vi "enable channel groups.vi"(8 "error in":errorcluster, 9 "Disable channel group?":bool[](array[boolean]), 10 "class path":path, 11 "Application in":refnum<vi>) -> (0 "error out":errorcluster)   [LabVIEW 2013, in "FixedChannelTBModuleDecideFeatures.lvclass"]
uses:
  FixedChannelTBModuleDecideFeatures.lvclass
  <vilib>/Utility/traverseref.llb/TRef TravTarget.ctl
  <vilib>/Utility/traverseref.llb/VI Scripting - Traverse.lvlib
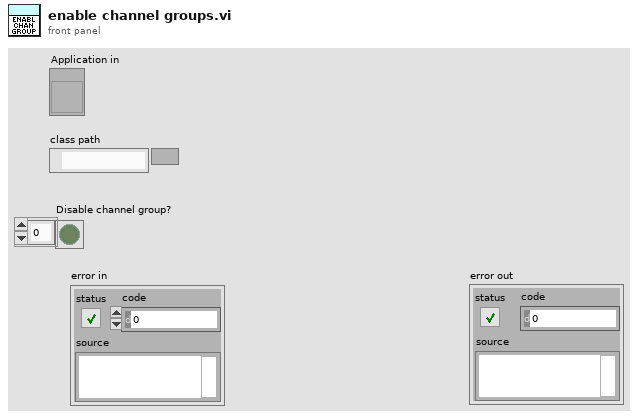
[diagram p1: front panel]
types:
  T1 = typedef "TRef TravTarget.ctl" = enum16{"FP", "BD", "Other"}
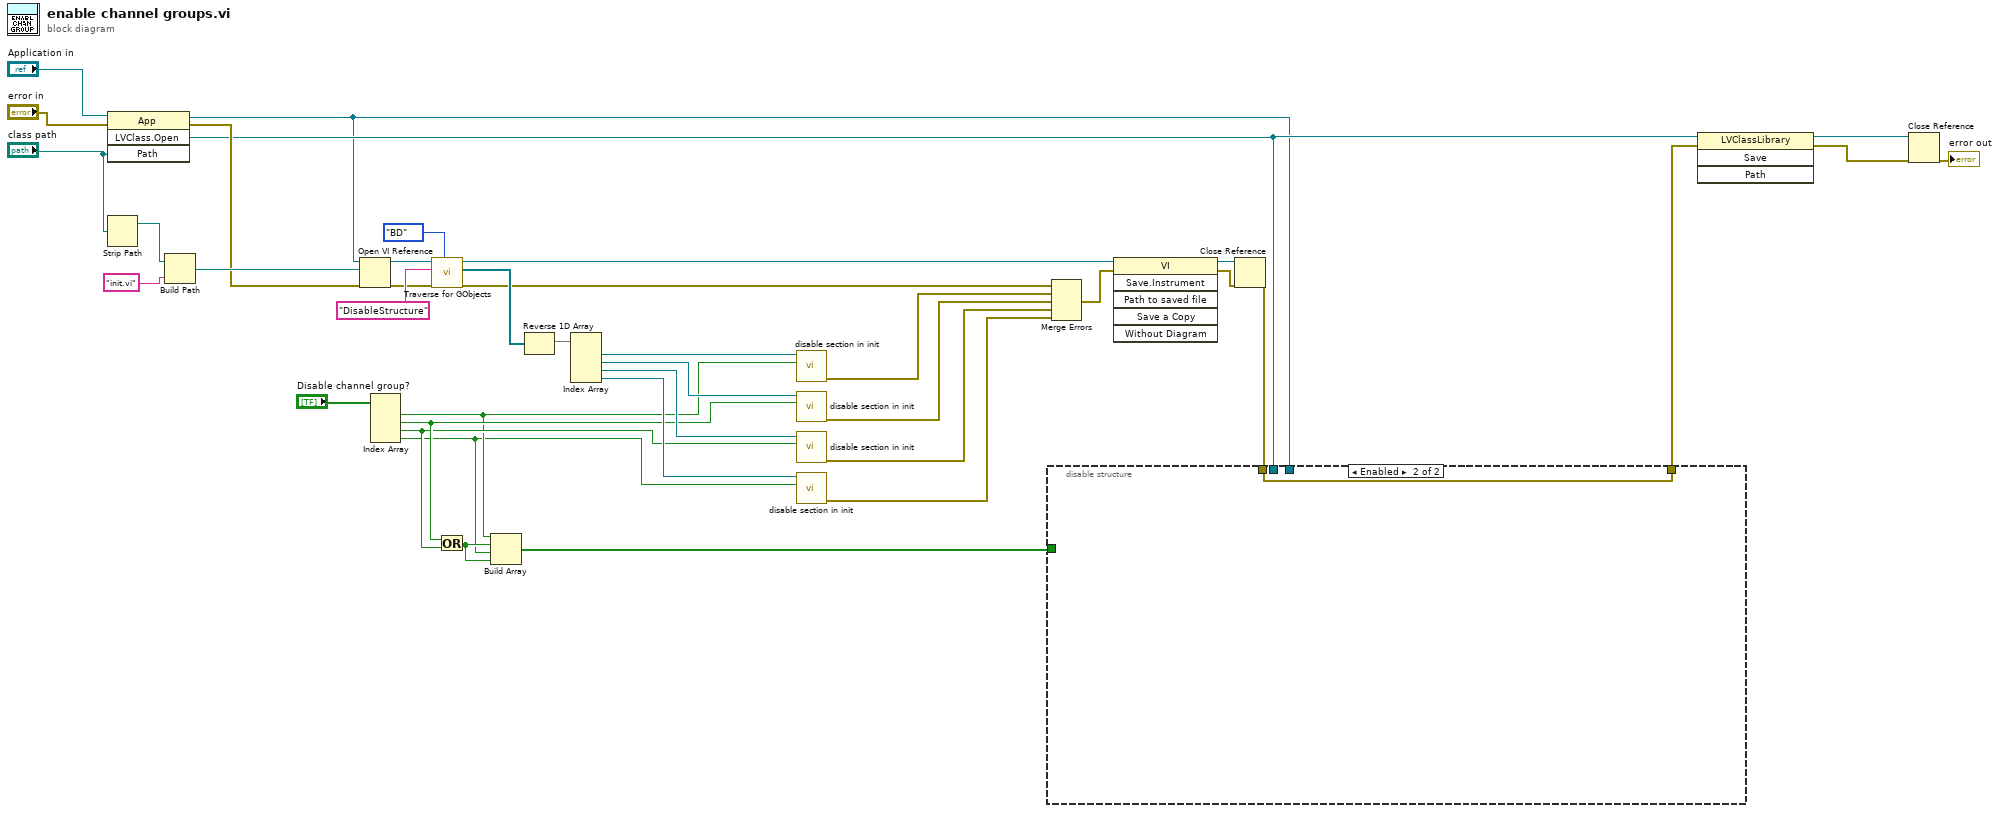
[diagram p0: block diagram]
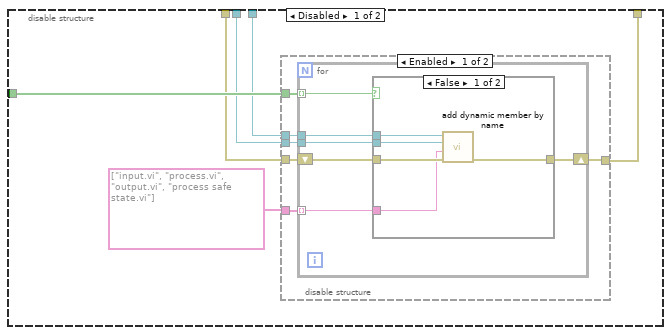
[diagram p2: hidden frame]
diagram:
  n1 = invoke class="App" method="LVClass.Open"(reference="Application in", error in="error in", "Path"="class path") -> (reference out=w1:refnum<vi>, error out=w12:errorcluster, "LVClass.Open"=w5:refnum<vi>)  [unwired: 1 in, 1 out]
  n2 = Strip Path(path="class path") -> (stripped path=w17:path)  [unwired: 1 out]
  n3 = Build Path(base path=w17, name or relative path="init.vi") -> (appended path=w15:path)
  n4 = Open VI Reference(application reference (local)=w1, vi path=w15, error in (no error)=w12) -> (vi reference=w14:refnum<vi>, error out=w11:errorcluster)  [unwired: 3 in]
  n5 = Index Array(array="Disable channel group?") -> (element #1=w26:bool, element #2=w29:bool, element #3=w28:bool, element #4=w25:bool)  [unwired: 4 in]
  n6 = call <vilib>:"Traverse for GObjects.vi"("Traverse Target"=TRef_TravTarget."BD", "error in (no error)"=w11, "Class Name"="DisableStructure", "VI Refnum"=w14) -> ("error out"=w10:errorcluster, "References"=w37:refnum<vi>[], "dup VI Refnum"=w34:refnum<vi>)  [unwired: 4 in, 1 out]
  n7 = Or(x=w29, y=w28) -> (x .or. y?=w27:bool)
  n8 = Build Array(w26, w27, w25, w27) -> (w24:bool[])
  n9 = Reverse 1D Array(array=w37) -> (reversed array=w36:refnum<vi>[])
  n10 = Index Array(array=w36) -> (element #1=w35:refnum<vi>, element #2=w32:refnum<vi>, element #3=w31:refnum<vi>, element #4=w30:refnum<vi>)  [unwired: 4 in]
  n11 = call "disable section in init.vi"("Boolean"=w26, "GObject in"=w35) -> ("error out"=w33:errorcluster)  [unwired: 9 in]
  n12 = call "disable section in init.vi"("Boolean"=w29, "GObject in"=w32) -> ("error out"=w22:errorcluster)  [unwired: 9 in]
  n13 = call "disable section in init.vi"("Boolean"=w28, "GObject in"=w31) -> ("error out"=w21:errorcluster)  [unwired: 9 in]
  n14 = call "disable section in init.vi"("Boolean"=w25, "GObject in"=w30) -> ("error out"=w13:errorcluster)  [unwired: 9 in]
  n15 = Merge Errors(w10, w33, w22, w21, w13) -> (w23:errorcluster)
  n16 = invoke class="VI" method="Save.Instrument"(reference=w34, error in=w23) -> (reference out=w8:refnum<vi>, error out=w9:errorcluster)  [unwired: 4 in, 4 out]
  n17 = Close Reference(reference=w8, error in (no error)=w9) -> (error out=w7:errorcluster)
  n18 = disable-structure shown="Enabled" {
    disable-tunnel: w24 -> [w46 _]
    disable-tunnel: w7 -> [w44 w66]
    disable-tunnel: w5 -> [w43 _]
    disable-tunnel: [w42 w66] -> w3
    disable-tunnel: w1 -> [w41 _]
    frame Disabled {
      n19 = disable-structure shown="Enabled" {
        disable-tunnel: w43 -> [w52 _]
        disable-tunnel: w46 -> [w51 _]
        disable-tunnel: string[] ["input.vi", "process.vi", "output.vi", "process safe state.vi"] -> [w50 _]
        disable-tunnel: w44 -> [w49 w65]
        disable-tunnel: [w48 w65] -> w42
        disable-tunnel: w41 -> [w47 _]
        frame Enabled {
          n20 = for {
            tunnel: w52 -> [w58]
            tunnel: w51 -> [w57] mode=indexing
            tunnel: w50 -> [w56] mode=indexing
            shift-right: [w55] -> w48
            shift-left: w49 -> [w54]
            tunnel: w47 -> [w53]
            n21 = case shown="False" w57 {
              tunnel: w58 -> [w61 _]
              tunnel: w56 -> [w60 _]
              tunnel: [w63 w64] -> w55
              tunnel: w54 -> [w62 w64]
              tunnel: w53 -> [w59 _]
              frame False {
                n22 = call "add dynamic member by name.vi"("error in (no error)"=w62, "name"=w60, "LVClassLibrary in"=w61, "Application in"=w59) -> ("error out"=w63:errorcluster)  [unwired: 7 in]
              }
              frame True {
              }
            }
          }
        }
        frame Disabled {
        }
      }
    }
    frame Enabled {
    }
  }
  n23 = invoke class="LVClassLibrary" method="Save"(reference=w5, error in=w3) -> (reference out=w4:refnum<vi>, error out=w2:errorcluster)  [unwired: 2 in, 2 out]
  n24 = Close Reference(reference=w4, error in (no error)=w2) -> (error out=→"error out":errorcluster)
